vi "Configure Math (Filter).vi"(0 "VISA resource name":refnum<visa-resource-name>, 7 "Filter type (0: And)":i32(ring) items=["High", "Low"], 9 "Channel (1)":i32(ring) items=["1", "2", "3", "4"], 11 "error in (no error)":errorcluster, 12 "Frequency (0)":dbl=10000.0) -> (4 "VISA resource name out":refnum<visa-resource-name>, 15 "error out":errorcluster)   [LabVIEW 2015, in "ZhiYuan ZDS Series for TCP.lvlib"]
doc: "Configures the setting for logic operation."
uses:
  ZhiYuan ZDS Series for TCP.lvlib
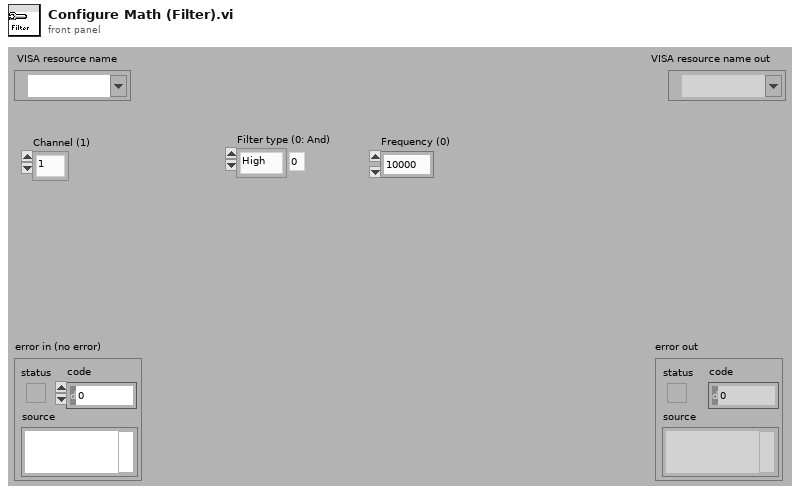
[diagram p1: front panel]
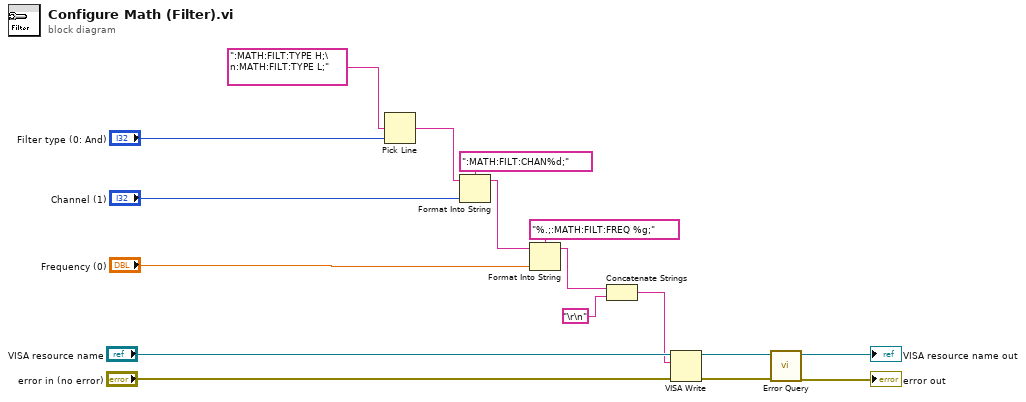
[diagram p0: block diagram]
diagram:
  n1 = Pick Line(multi-line string=":MATH:FILT:TYPE H;\n:MATH:FILT:TYPE L;", line index="Filter type (0: And)") -> (output string=w15:string)  [unwired: 1 in]
  n2 = Format Into String(format string=":MATH:FILT:CHAN%d;", initial string=w15, "Channel (1)") -> (resulting string=w4:string)  [unwired: 1 in, 1 out]
  n3 = Format Into String(format string="%.;:MATH:FILT:FREQ %g;", initial string=w4, "Frequency (0)") -> (resulting string=w3:string)  [unwired: 1 in, 1 out]
  n4 = Concatenate Strings(w3, "\r\n") -> (w1:string)
  n5 = VISA Write(VISA resource name="VISA resource name", write buffer=w1, error in (no error)="error in (no error)") -> (VISA resource name out=w8:refnum<visa-resource-name>, error out=w7:errorcluster)  [unwired: 1 out]
  n6 = call "Error Query.vi"("error in (no error)"=w7, "VISA resource name"=w8) -> ("error out"=→"error out":errorcluster, "VISA resource name out"=→"VISA resource name out":refnum<visa-resource-name>)  [unwired: 6 in, 2 out]
